vi "enableAllInstrumentErrors.vi"(8 "error in (no error)":errorcluster, 11 "Electrometer in":refnum<class "Electrometer.lvclass">) -> (0 "error out":errorcluster, 3 "Electrometer out":refnum<class "Electrometer.lvclass">)   [LabVIEW 2016, in "Electrometer.lvclass"]
uses:
  Electrometer.lvclass
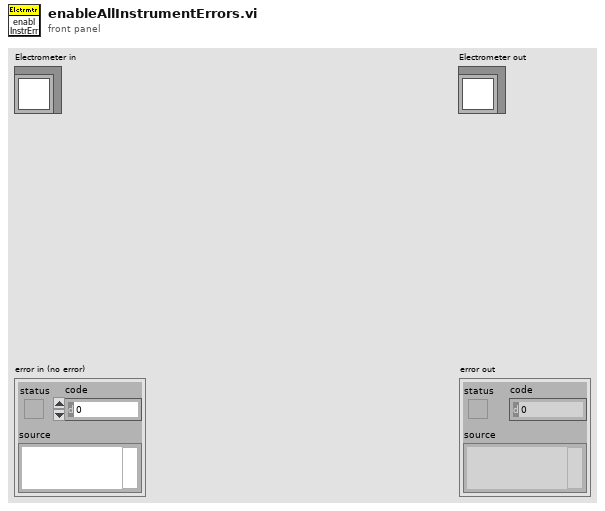
[diagram p1: front panel]
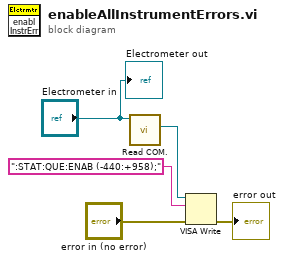
[diagram p0: block diagram]
diagram:
  n1 = call "Read COM..vi"("Electrometer in"="Electrometer in") -> ("VISA"=w1:refnum<visa-resource-name>)  [unwired: 8 in, 2 out]
  n2 = VISA Write(VISA resource name=w1, write buffer=":STAT:QUE:ENAB (-440:+958);", error in (no error)="error in (no error)") -> (error out=→"error out":errorcluster)  [unwired: 2 out]
  "Electrometer out" <- "Electrometer in"
